vi "Cluster to Array.vi"(1 "Data Struct - All":T1) -> (0 "Output Array":string[](array[string]))   [LabVIEW 2020]
uses:
  Control/Data Struct - All.ctl
  Control/Data Struct - SB.ctl
  Control/Data Struct - Bank.ctl
  Control/Data Struct - SI.ctl
  Control/Data Struct - PM.ctl
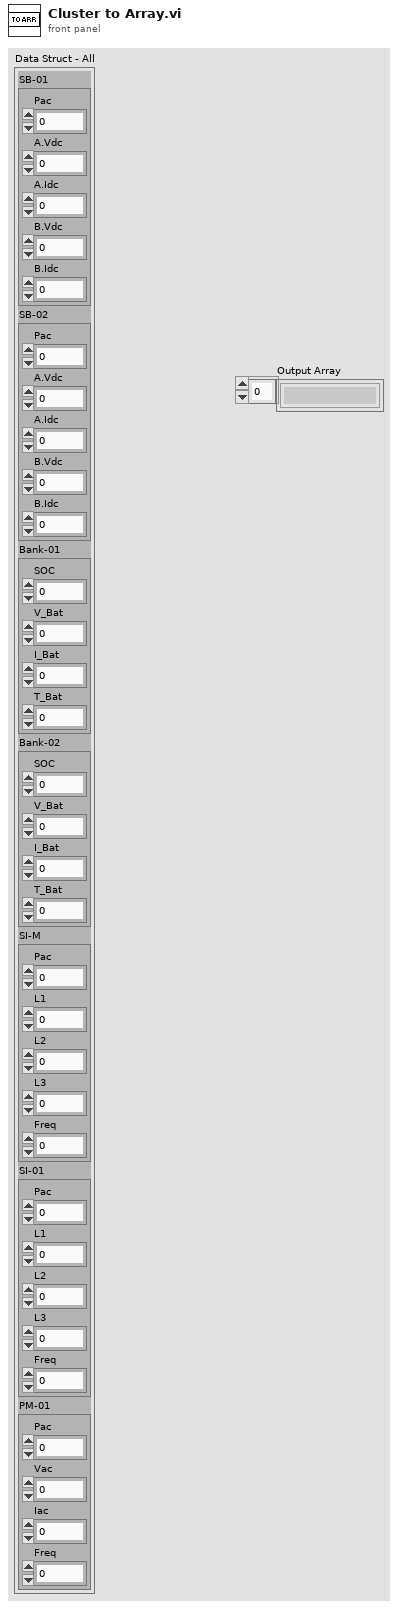
[diagram p1: front panel]
types:
  T1 = typedef "Data Struct - All.ctl" = cluster{"SB-01":T2, "SB-02":T2, "Bank-01":T3, "Bank-02":T3, "SI-M":T4, "SI-01":T4, "PM-01":T5}
  T2 = typedef "Data Struct - SB.ctl" = cluster{"Pac":dbl, "A.Vdc":dbl, "A.Idc":dbl, "B.Vdc":dbl, "B.Idc":dbl}
  T3 = typedef "Data Struct - Bank.ctl" = cluster{"SOC":dbl, "V_Bat":dbl, "I_Bat":dbl, "T_Bat":dbl}
  T4 = typedef "Data Struct - SI.ctl" = cluster{"Pac":dbl, "L1":dbl, "L2":dbl, "L3":dbl, "Freq":dbl}
  T5 = typedef "Data Struct - PM.ctl" = cluster{"Pac":dbl, "Vac":dbl, "Iac":dbl, "Freq":dbl}
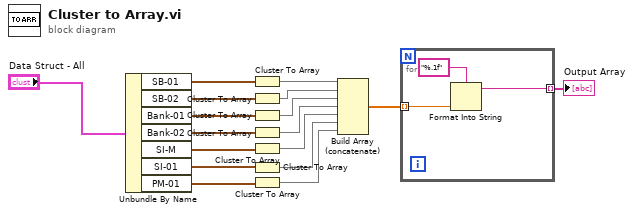
[diagram p0: block diagram]
diagram:
  n1 = Unbundle By Name("Data Struct - All") -> ("SB-01"=w16:T2, "SB-02"=w15:T2, "Bank-01"=w14:T3, "Bank-02"=w13:T3, "SI-M"=w12:T4, "SI-01"=w11:T4, "PM-01"=w10:T5)
  n2 = Cluster To Array(cluster=w16) -> (array=w9:dbl[])
  n3 = Cluster To Array(cluster=w15) -> (array=w8:dbl[])
  n4 = Cluster To Array(cluster=w14) -> (array=w7:dbl[])
  n5 = Cluster To Array(cluster=w13) -> (array=w6:dbl[])
  n6 = Cluster To Array(cluster=w12) -> (array=w5:dbl[])
  n7 = Cluster To Array(cluster=w11) -> (array=w4:dbl[])
  n8 = Cluster To Array(cluster=w10) -> (array=w3:dbl[])
  n9 = Build Array (concatenate)(w9, w8, w7, w6, w5, w4, w3) -> (w2:dbl[])
  n10 = for {
    tunnel: w2 -> [w20] mode=indexing
    tunnel: [w18] -> w1 mode=indexing
    n11 = Format Into String(format string="%.1f", w20) -> (resulting string=w18:string)  [unwired: 2 in, 1 out]
  }
  "Output Array" <- w1
